vi "Test Report Contain Format Definition.vi"(8 "error in (no error)":errorcluster, 11 "XML Report Test in":refnum<class "XML Report Test.lvclass">) -> (0 "error out":errorcluster, 3 "XML Report Test out":refnum<class "XML Report Test.lvclass">)   [LabVIEW 2020, in "XML Report Test.lvclass"]
uses:
  XML Report Test.lvclass
  source/Plugins/XML Report/XML Report.lvclass
  XML Report Test.lvclass/XML Report Test.ctl
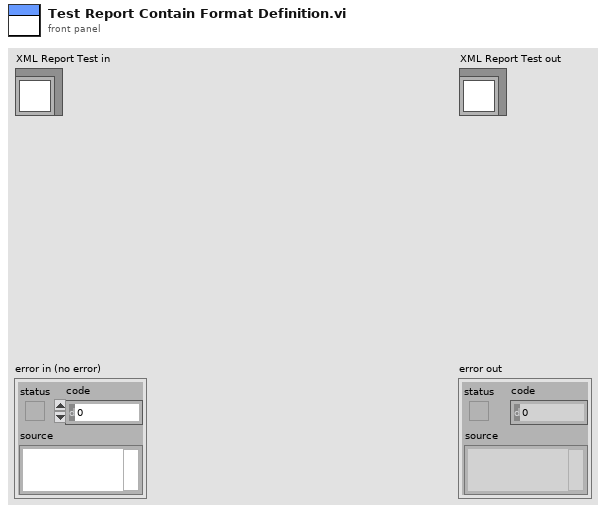
[diagram p1: front panel]
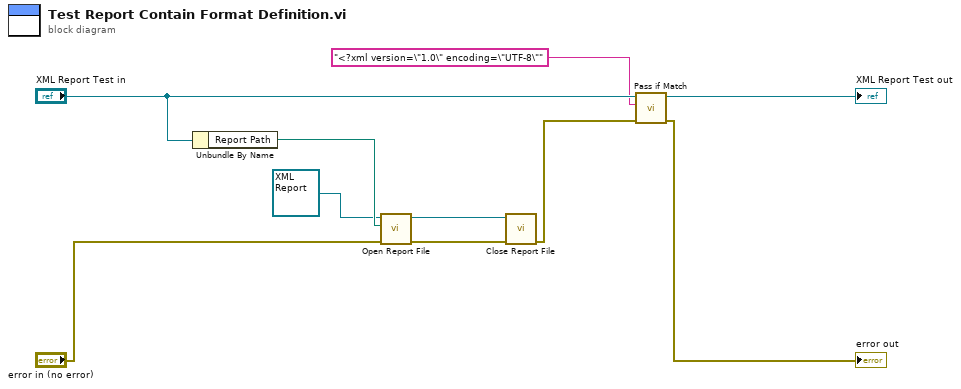
[diagram p0: block diagram]
diagram:
  n1 = Unbundle By Name("XML Report Test in") -> ("Report Path"=w3:path)
  n2 = call-dynamic "Open Report File.vi"("error in (no error)"="error in (no error)", "Report Path"=w3, "XML Report In"=refnum<class "XML Report.lvclass"> refnum) -> ("error out"=w10:errorcluster, "XML Report Out"=w9:refnum<class "XML Report.lvclass">)  [unwired: 7 in]
  n3 = call-dynamic "Close Report File.vi"("error in (no error)"=w10, "XML Report In"=w9) -> ("error out"=w5:errorcluster)  [unwired: 9 in]
  n4 = call "Pass if Match.vi"("error in (no error)"=w5, "regular expression"="<?xml version=\"1.0\" encoding=\"UTF-8\"", "XML Report Test in"="XML Report Test in") -> ("error out"=→"error out":errorcluster, "XML Report Test out"=→"XML Report Test out":refnum<class "XML Report Test.lvclass">)  [unwired: 7 in]
